vi "CalculateSpacing.vi"(2 "Scan Type":enum8{"Circular", "Square", "Hexagonal"}(ring), 3 "Points per Scan":u8, 4 "Radius (V)":dbl) -> (0 "Maximum Voltage (V)":dbl, 1 "Spacing (V)":dbl)   [LabVIEW 2011]
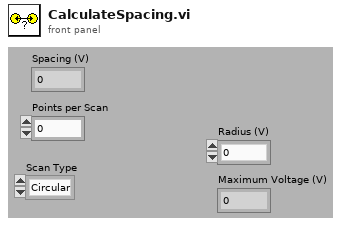
[diagram p1: front panel]
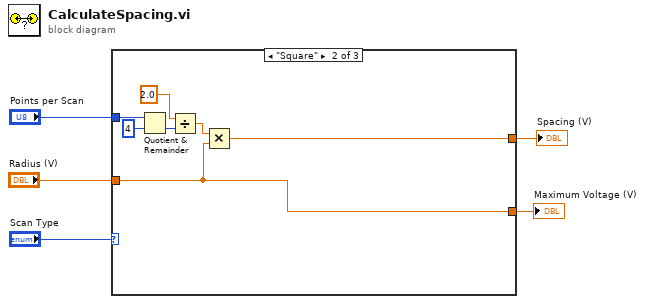
[diagram p0: block diagram]
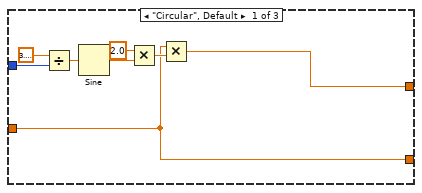
[diagram p2: hidden frame]
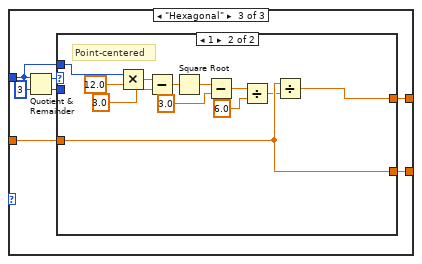
[diagram p3: hidden frame]
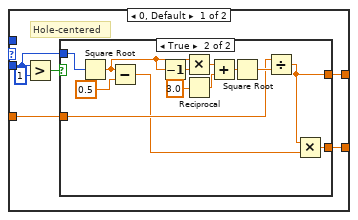
[diagram p4: hidden frame]
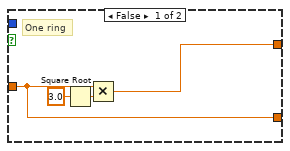
[diagram p5: hidden frame]
diagram:
  n1 = case shown="\"Square\"" "Scan Type" {
    tunnel: "Points per Scan" -> [w9 w20 w21]
    tunnel: "Radius (V)" -> [w6 w14 w24]
    tunnel: [w7 w17 w23] -> w1
    tunnel: [w6 w14 w22] -> w3
    frame "Circular", Default {
      n2 = Divide(x=3.141592653589793, y=w9) -> (x/y=w12:dbl)
      n3 = Sine(x=w12) -> (sin(x)=w11:dbl)
      n4 = Multiply(x=2.0, y=w11) -> (x*y=w8:dbl)
      n5 = Multiply(x=w6, y=w8) -> (x*y=w7:dbl)
    }
    frame "Square" {
      n6 = Quotient & Remainder(x=w20, y=u8 4) -> (floor(x/y)=w15:u8)  [unwired: 1 out]
      n7 = Divide(x=2.0 ("y"), y=w15) -> (x/y=w18:dbl)
      n8 = Multiply(x=w18, y=w14) -> (x*y=w17:dbl)
    }
    frame "Hexagonal" {
      n9 = Quotient & Remainder(x=w21, y=u8 3) -> (x-y*floor(x/y)=w26:u8, floor(x/y)=w25:u8)
      n10 = case shown="1" w26 {
        tunnel: w25 -> [w28 _]
        tunnel: w24 -> [w31 w52]
        tunnel: [w30 w53] -> w23
        tunnel: [w29 w52] -> w22
        tunnel: w21 -> [_ w62]
        frame 0, Default {
          # "Hole-centered"
          n11 = Greater?(x=w28, y=u8 1) -> (0:w32:bool)
          n12 = case shown="True" w32 {
            tunnel: w31 -> [w34 w40]
            tunnel: [w35 w39] -> w30
            tunnel: [w34 w48] -> w29
            tunnel: w28 -> [_ w50]
            frame False {
              # "One ring"
              n13 = Square Root(x=3.0) -> (sqrt(x)=w37:dbl)
              n14 = Multiply(x=w34, y=w37) -> (x*y=w35:dbl)
            }
            frame True {
              n15 = Square Root(x=w50) -> (sqrt(x)=w46:dbl)
              n16 = Subtract(x=w46, y=0.5) -> (x-y=w38:dbl)
              n17 = Decrement(x=w46) -> (x-1=w47:dbl)
              n18 = Multiply(x=w46, y=w47) -> (x*y=w45:dbl)
              n19 = Reciprocal(x=3.0) -> (1/x=w44:dbl)
              n20 = Add(x=w45, y=w44) -> (x+y=w42:dbl)
              n21 = Square Root(x=w42) -> (sqrt(x)=w41:dbl)
              n22 = Divide(x=w40, y=w41) -> (x/y=w39:dbl)
              n23 = Multiply(x=w39, y=w38) -> (x*y=w48:dbl)
            }
          }
        }
        frame 1 {
          # "Point-centered"
          n24 = Multiply(x=w62, y=12.0) -> (x*y=w60:dbl)
          n25 = Subtract(x=w60, y=3.0) -> (x-y=w58:dbl)
          n26 = Square Root(x=w58) -> (sqrt(x)=w57:dbl)
          n27 = Subtract(x=w57, y=3.0) -> (x-y=w55:dbl)
          n28 = Divide(x=w55, y=6.0) -> (x/y=w51:dbl)
          n29 = Divide(x=w52, y=w51) -> (x/y=w53:dbl)
        }
      }
    }
  }
  "Spacing (V)" <- w1
  "Maximum Voltage (V)" <- w3
